vi "Run Bfr Tx - Check Transmit.vi"(8 "error in (no error)":errorcluster, 11 "Tx Loop Data in":T1 {"Data Buffer" format="%016x"}) -> (0 "error out":errorcluster, 1 "Bytes to Transmit":i32, 2 "Transmit?":bool, 3 "Tx Loop Data out":T1 {"Data Buffer" format="%016x"})   [LabVIEW 2016, in "UDP-Custom-Device Engine.lvlib"]
uses:
  UDP-Custom-Device Engine.lvlib
  Types/Engine - Buffered Tx Loop Data.ctl
  Shared/Types/Shared - Header Details.ctl
  Shared/Types/Shared - Buffered.PacketInfo.ctl
  <vilib>/NI/NIVS Inline Async API/_Data Access Engine/Data Access Engine/Types/ReadWrite.DVR.ctl
  <vilib>/NI/NIVS Inline Async API/_Data Access Engine/Access Type Classes/ReadWrite/ReadWrite.lvclass
  <vilib>/NI/NIVS Inline Async API/_Data Access Engine/Data Access Engine/Types/Read.DVR.ctl
  <vilib>/NI/NIVS Inline Async API/_Data Access Engine/Access Type Classes/Read/Read.lvclass
  <vilib>/NI/NIVS Inline Async API/_Data Access Engine/Data Access Engine/Types/Write.DVR.ctl
  <vilib>/NI/NIVS Inline Async API/_Data Access Engine/Access Type Classes/Write/Write.lvclass
  Shared/Types/Shared - Duplex Settings.ctl
  <vilib>/NI/NIVS Inline Async API/_Data Access Engine/Access Type Classes/ReadWrite/ReadWrite.lvclass/ReadWrite.ctl
  <vilib>/NI/NIVS Inline Async API/_Data Access Engine/Access Type Classes/Read/Read.lvclass/Read.ctl
  <vilib>/NI/NIVS Inline Async API/_Data Access Engine/Data Access Engine/Methods/ReadWrite.Data.vi
  <vilib>/NI/NIVS Inline Async API/_Data Access Engine/Data Access Engine/Methods/Read.Data.vi
  <vilib>/NI Veristand/VeriStand Data/Library/Type Conversion/Type Conversion.From Double (I32).vi
  <vilib>/NI/NIVS Inline Async API/_Data Access Engine/Access Type Classes/ReadWrite/ReadWrite.ProcessData.vi
  <vilib>/NI/NIVS Inline Async API/_Data Access Engine/Access Type Classes/Read/Read.ProcessData.vi
  <vilib>/NI/NIVS Inline Async API/_Data Access Engine/Data Access Engine/Data Access Engine.lvclass
  <vilib>/NI Veristand/VeriStand Data/Library/VeriStand Data.lvlib
  Shared/UDP-Custom-Device Shared.lvlib
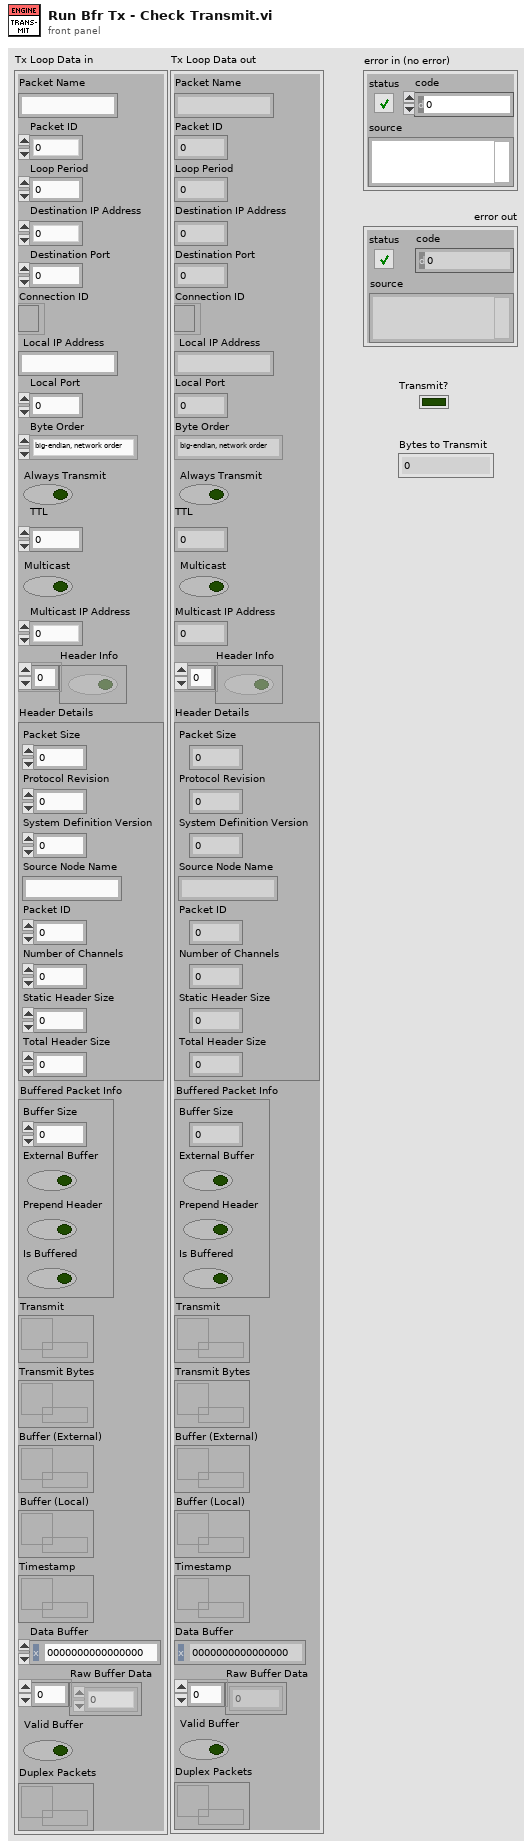
[diagram p1: front panel]
types:
  T1 = typedef "UDP-Custom-Device Engine.lvlib/Engine - Buffered Tx Loop Data.ctl" = cluster{"Packet Name":string, "Packet ID":i32, "Loop Period":u32, "Destination IP Address":u32, "Destination Port":u16, "Connection ID":refnum<k16>, "Local IP Address":string, "Local Port":i32, "Byte Order":enum16{"big-endian, network order", "native, host order", "little-endian"}, "Always Transmit":bool, "TTL":u16, "Multicast":bool, "Multicast IP Address":u32, "Header Info":bool[], "Header Details":T2, "Buffered Packet Info":T3, "Transmit":T4, "Transmit Bytes":T5, "Buffer (External)":T5, "Buffer (Local)":T6, "Timestamp":T5, "Data Buffer":u64, "Raw Buffer Data":u8[], "Valid Buffer":bool, "Duplex Packets":refnum<data-value>}
  T2 = typedef "UDP-Custom-Device Shared.lvlib/Shared - Header Details.ctl" = cluster{"Packet Size":u16, "Protocol Revision":u8, "System Definition Version":u64, "Source Node Name":string, "Packet ID":u32, "Number of Channels":u32, "Static Header Size":u16, "Total Header Size":u16}
  T3 = typedef "UDP-Custom-Device Shared.lvlib/Shared - Buffered.PacketInfo.ctl" = cluster{"Buffer Size":i32, "External Buffer":bool, "Prepend Header":bool, "Is Buffered":bool}
  T4 = typedef "Data Access Engine.lvlib/Data Access Engine.lvclass/ReadWrite.DVR.ctl" = refnum<data-value>
  T5 = typedef "Data Access Engine.lvlib/Data Access Engine.lvclass/Read.DVR.ctl" = refnum<data-value>
  T6 = typedef "Data Access Engine.lvlib/Data Access Engine.lvclass/Write.DVR.ctl" = refnum<data-value>
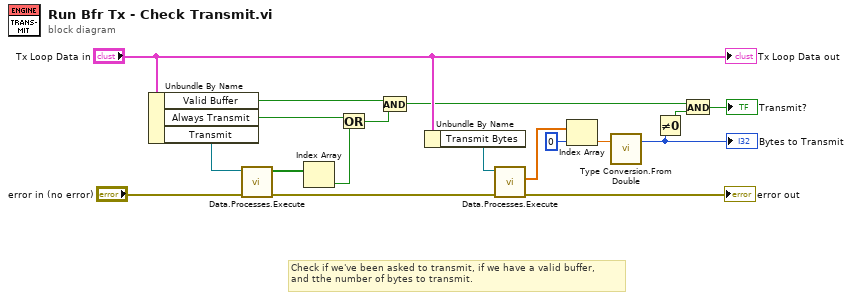
[diagram p0: block diagram]
diagram:
  # "Check if we've been asked to transmit, if we have a valid buffer,\nand tthe number of bytes to transmit."
  n1 = Unbundle By Name("Tx Loop Data in") -> ("Valid Buffer"=w10:bool, "Always Transmit"=w18:bool, "Transmit"=w4:T4)
  n2 = call-poly <vilib>:"Data.Processes.Execute.vi"("error in (no error)"="error in (no error)", "Ref"=w4) -> ("error out"=w3:errorcluster, "Detect?"=w2:bool[])  [unwired: 6 in, 2 out]
  n3 = Index Array(array=w2) -> (element=w1:bool)  [unwired: 1 in]
  n4 = Or(x=w18, y=w1) -> (x .or. y?=w17:bool)
  n5 = And(x=w10, y=w17) -> (x .and. y?=w7:bool)
  n6 = Unbundle By Name("Tx Loop Data in") -> ("Transmit Bytes"=w16:T5)
  n7 = call-poly <vilib>:"Data.Processes.Execute.vi"("error in (no error)"=w3, "Ref"=w16) -> ("error out"=→"error out":errorcluster, "Values"=w14:dbl[])  [unwired: 7 in, 1 out]
  n8 = Index Array(array=w14, index=0) -> (element=w12:dbl)
  n9 = call-poly <vilib>:"Type Conversion.From Double.vi"("value in"=w12) -> ("value out"=w8:i32)  [unwired: 2 in]
  "Bytes to Transmit" <- w8
  n10 = Not Equal To 0?(x=w8) -> (x != 0?=w5:bool)
  n11 = And(x=w7, y=w5) -> (x .and. y?=→"Transmit?":bool)
  "Tx Loop Data out" <- "Tx Loop Data in"
